vi "BM_scpi_sr_test.vi"() -> ()   [LabVIEW 2009]
panel:
  out "Error out":errorcluster
  in  "error in (no error)":errorcluster
  out "Reply":string
  in  "Command":string="rout:chan:verify:pos:state? (@5101)\n"
  in  "Instrument":T1(ring)=enum."34980a"
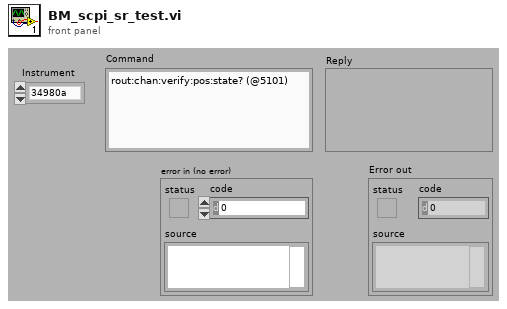
[diagram p1: front panel]
types:
  T1 = enum16{"N1911A", "Siggen", "34980a", "E4418B", "Rvp8"}
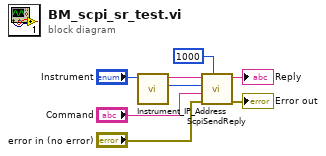
[diagram p0: block diagram]
diagram:
  n1 = call "Instrument_IP_Address.vi"("Instrument"="Instrument") -> ("Port"=w7:u16, "IP Address"=w8:string)  [unwired: 9 in]
  n2 = call "ScpiSendReply.vi"("TCP Timeout mS"=1000, "error in (no error)"="error in (no error)", "Command"="Command", "TCP port"=w7, "IP Address"=w8) -> ("Error out"=→"Error out":errorcluster, "Reply"=→"Reply":string)  [unwired: 4 in]
